vi "Add New Step.vi"(8 "Error In":errorcluster, 9 "Duration (s)":dbl, 10 "Fire (%)":dbl, 11 "reference in":refnum<class "Recipe.lvclass">) -> (0 "Error Out":errorcluster, 3 "reference out":refnum<class "Recipe.lvclass">)   [LabVIEW 2024, in "Recipe.lvclass"]
uses:
  Recipe.lvclass
  Recipe Step/Recipe Step.lvclass
  Recipe.lvclass/Recipe.ctl
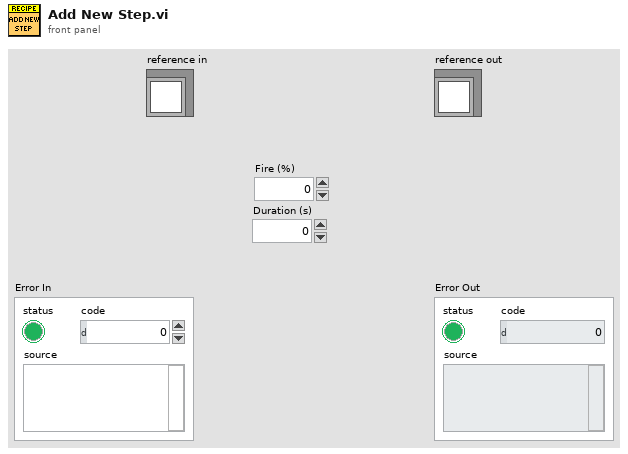
[diagram p1: front panel]
types:
  T1 = typedef "Recipe.lvclass/ObjectAttributes.ctl" = cluster{"Steps":refnum<class "Recipe Step.lvclass">[], "Current Info":cluster{"Current Index":u64}}
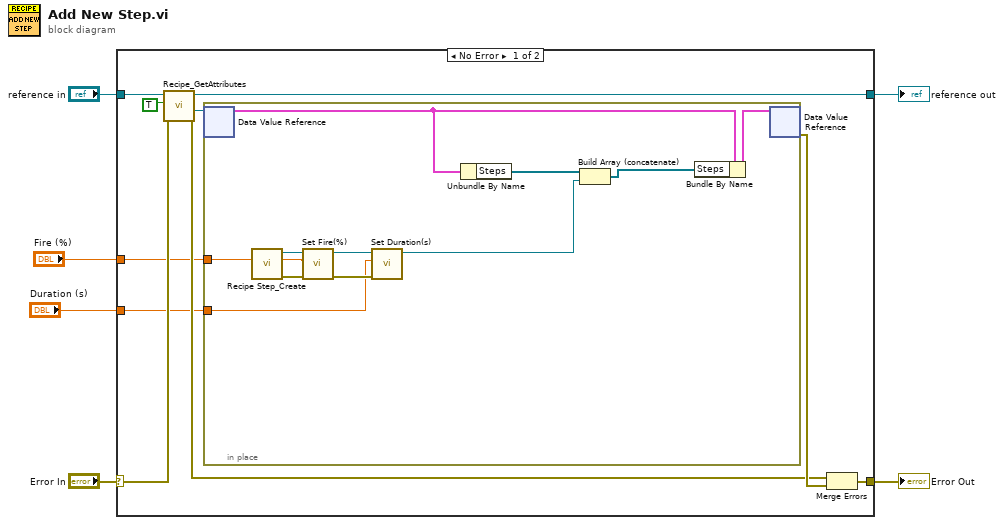
[diagram p0: block diagram]
diagram:
  n1 = case shown="No Error" "Error In" {
    selector: "Error In" -> [w14 w29]
    tunnel: [w9 w29] -> w5
    tunnel: [w15 w28] -> w3
    tunnel: "reference in" -> [w16 w28]
    tunnel: "Fire (%)" -> [w8 _]
    tunnel: "Duration (s)" -> [w7 _]
    frame No Error {
      n2 = call "Recipe_GetAttributes.vi"("Error In"=w14, "OnlyGetDvrReference(False)"=TRUE, "reference in"=w16) -> ("Error Out"=w10:errorcluster, "DataRef"=w11:refnum<data-value>, "reference out"=w15:refnum<class "Recipe.lvclass">)  [unwired: 5 in, 1 out]
      n3 = in-place {
        in-place-border: w8 -> [w24]
        in-place-border: w7 -> [w23]
        n4 = in-place-dvr #1(w11) -> (w22:T1)  [unwired: 1 out]
        n5 = call "Recipe Step_Create.vi"() -> ("Error Out"=w18:errorcluster, "reference out"=w17:refnum<class "Recipe Step.lvclass">)  [unwired: 10 in]
        n6 = call-dynamic "Set Fire(%).vi"("Error In"=w18, "Fire (%)"=w24, "reference in"=w17) -> ("Error Out"=w26:errorcluster, "reference out"=w25:refnum<class "Recipe Step.lvclass">)  [unwired: 7 in]
        n7 = call-dynamic "Set Duration(s).vi"("Error In"=w26, "Duration (s)"=w23, "reference in"=w25) -> ("reference out"=w19:refnum<class "Recipe Step.lvclass">)  [unwired: 7 in, 1 out]
        n8 = Unbundle By Name(w22) -> ("Steps"=w21:refnum<class "Recipe Step.lvclass">[])
        n9 = Build Array (concatenate)(w21, w19) -> (w20:refnum<class "Recipe Step.lvclass">[])
        n10 = Bundle By Name(cluster=w22, "Steps"=w20) -> (w27:T1)
        n11 = in-place-dvr #1(w27) -> (w12:errorcluster)  [unwired: 1 out]
      }
      n12 = Merge Errors(w10, w12) -> (w9:errorcluster)
    }
    frame Error {
    }
  }
  "Error Out" <- w5
  "reference out" <- w3
